vi "find_vmp_from_log.vi"(7 "Cell details cluster in":T1, 11 "File path of JV log":path) -> (3 "Vmp":dbl)   [LabVIEW 2016]
uses:
  <vilib>/Utility/file.llb/Read From Spreadsheet File (string).vi
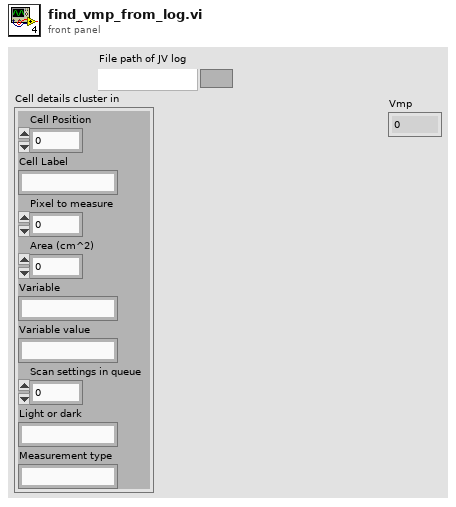
[diagram p1: front panel]
types:
  T1 = cluster{"Cell Position":i32, "Cell Label":string, "Pixel to measure":u16, "Area (cm^2)":dbl, "Variable":string, "Variable value":string, "Scan settings in queue":u16, "Light or dark":string, "Measurement type":string}
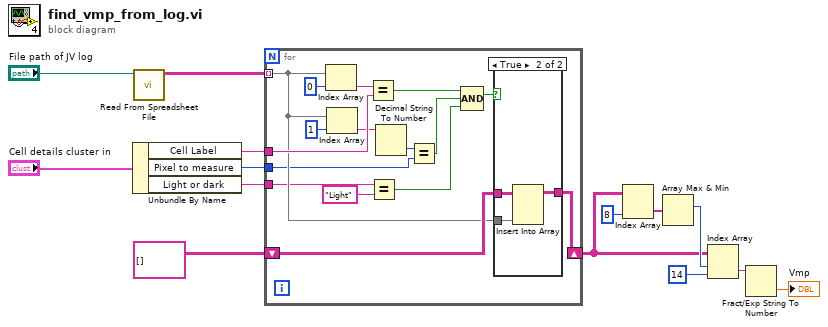
[diagram p0: block diagram]
diagram:
  n1 = Unbundle By Name("Cell details cluster in") -> ("Cell Label"=w12:string, "Pixel to measure"=w3:u16, "Light or dark"=w2:string)
  n2 = call-poly <vilib>:"Read From Spreadsheet File.vi"("file path (dialog if empty)"="File path of JV log") -> ("all rows"=w13:string[][])  [unwired: 6 in, 4 out]
  n3 = for {
    tunnel: w13 -> [w25] mode=indexing
    tunnel: w12 -> [w28]
    shift-right: [w26] -> w7
    shift-left: string[][] [] ("all rows") -> [w27]
    tunnel: w3 -> [w21]
    tunnel: w2 -> [w17]
    n4 = Index Array(array=w25, index=0) -> (element=w29:string)
    n5 = Index Array(array=w25, index=1) -> (element=w23:string)
    n6 = Equal?(x=w29, y=w28) -> (x = y?=w19:bool)
    n7 = Equal?(x=w17, y="Light") -> (x = y?=w15:bool)
    n8 = Decimal String To Number(string=w23) -> (number=w22:i32)  [unwired: 2 in, 1 out]
    n9 = Equal?(x=w22, y=w21) -> (x = y?=w18:bool)
    n10 = Compound Arithmetic op=AND(w19, w18, w15) -> (w20:bool)
    n11 = case shown="True" w20 {
      tunnel: w27 -> [w31 w34]
      tunnel: [w31 w33] -> w26
      tunnel: w25 -> [_ w32]
      frame False {
      }
      frame True {
        n12 = Insert Into Array(array=w34, new element=w32) -> (w33:string[][])  [unwired: 2 in]
      }
    }
  }
  n13 = Index Array(array=w7, index (col)=8 ("disabled index (col)")) -> (element=w9:string[])  [unwired: 1 in]
  n14 = Array Max & Min(array=w9) -> (max index (indices)=w8:i32)  [unwired: 3 out]
  n15 = Index Array(array=w7, index (row)=w8, index (col)=14 ("disabled index (col)")) -> (element=w4:string)
  n16 = Fract/Exp String To Number(string=w4) -> (number=→"Vmp":dbl)  [unwired: 3 in, 1 out]
